vi "Drivetrain.vi"() -> ()   [LabVIEW 2012]
uses:
  <vilib>/Rock Robotics/WPI/Solenoid/WPI_SolenoidValue.ctl
  Robot Global Data.vi
  <vilib>/Rock Robotics/WPI/RobotDrive/WPI_RobotDriveGetSetRefNum.vi
  <vilib>/addons/control/pid/NI_PID_pid.lvlib
  <vilib>/addons/control/pid/pid.llb/PID (DBL).vi
panel:
  in  "PID gains":T1={"proportional gain (Kc)"=20.0, "integral time (Ti, min)"=0.008, "derivative time (Td, min)"=0.001} {"derivative time (Td, min)" format="%.3f"; "integral time (Ti, min)" format="%.3f"; "proportional gain (Kc)" format="%.3f"}
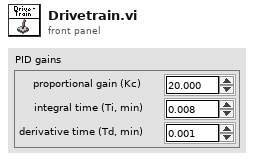
[diagram p1: front panel]
types:
  T1 = cluster{"proportional gain (Kc)":dbl, "integral time (Ti, min)":dbl, "derivative time (Td, min)":dbl}
  T2 = typedef "WPI_SolenoidValue.ctl" = enum16{"Off", "On", "Forward", "Reverse"}
  T3 = typedef "WPI_RelayDevRef.ctl" = cluster{"DevStatus":errorcluster, "Relay Channel":T4, "Digital Module":T5, "Relay Direction":T6}
  T4 = typedef "FPGA_DIORelayChannel.ctl" = enum8{"Relay 1", "Relay 2", "Relay 3", "Relay 4", "Relay 5", "Relay 6", "Relay 7", "Relay 8", "Invalid"}
  T5 = typedef "FPGA_TypedefDigitalModule.ctl" = enum16{"Digital Module 1", "Digital Module 2"}
  T6 = typedef "WPI_RelayDirection.ctl" = enum16{"Both directions", "Forward only", "Reverse only"}
  T7 = typedef "WPI_RobotDriveDevRef.ctl" = cluster{"DevStatus":errorcluster, "Motors[]":T8[], "Square Inputs":bool, "Max Output":dbl, "Isochronous":bool}
  T8 = typedef "WPI_MotorControlDeviceRef.ctl" = cluster{"DeviceStatus":errorcluster, "Type":enum16{"PWM", "CAN"}, "PWM":cluster{"Digital Module":T5, "PWM Channel":T9, "DeadBand":T10}, "CAN":cluster{"Device Number":u8, "Control Mode":T11, "Semaphore":T12, "Max Vout":dbl}, "Invert":bool, "TransformRef":T13, "InvTransformRef":T13}
  T9 = typedef "FPGA_DIOPWMChannel.ctl" = enum8{"PWM 1", "PWM 2", "PWM 3", "PWM 4", "PWM 5", "PWM 6", "PWM 7", "PWM 8", "PWM 9", "PWM 10", "Invalid"}
  T10 = typedef "WPI_PWMDeadband.ctl" = cluster{"Name":string, "maxPositivePwm":i32, "minPositivePwm":i32, "centerPwm":i32, "maxNegativePwm":i32, "minNegativePwm":i32, "angularRange":u16}
  T11 = typedef "WPI_CANJaguar_ControlMode.ctl" = enum8{"Percent VBus", "Current", "Speed", "Position", "Voltage"}
  T12 = typedef "Semaphore RefNum" = refnum<k1>
  T13 = typedef "WPI_PWMTransform_ConPane.ctl" = refnum<vi>
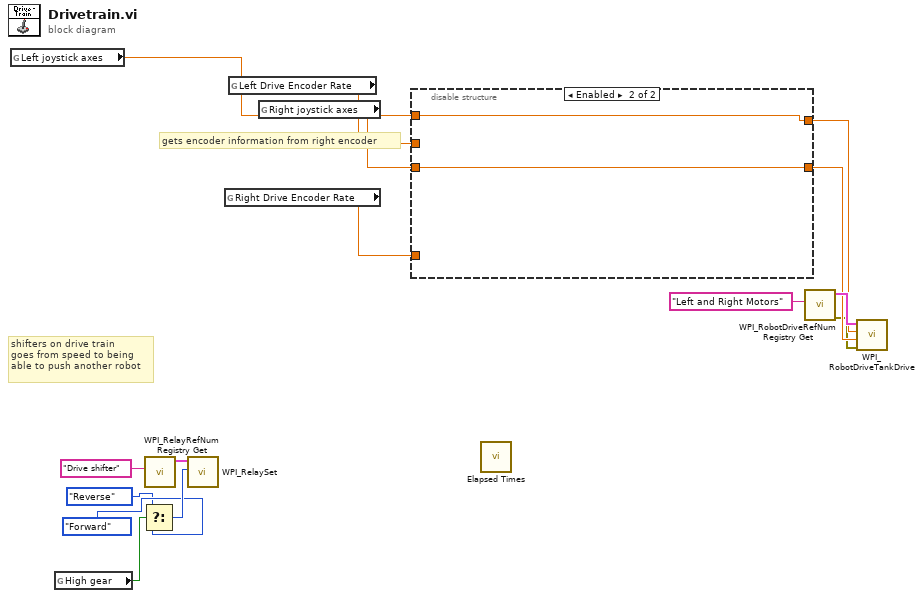
[diagram p0: block diagram]
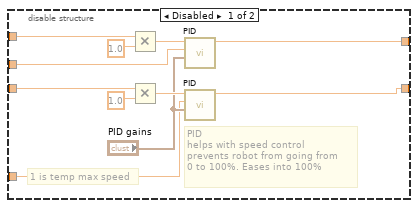
[diagram p2: hidden frame]
diagram:
  # "shifters on drive train\ngoes from speed to being\nable to push another robot"
  # "gets encoder information from right encoder"
  n1 = global read "Robot Global Data.vi" "Left joystick axes"() -> (w8:dbl)
  n2 = global read "Robot Global Data.vi" "High gear"() -> (w5:bool)
  n3 = Select(t=WPI_SolenoidValue."Reverse" ("Value"), s=w5, f=WPI_SolenoidValue."Forward" ("Value")) -> (s? t:f=w6:T2)
  n4 = call <vilib>:"WPI_RelayRefNum Registry Get.vi"("refnum name"="Drive shifter") -> ("RelayDevRef"=w2:T3)  [unwired: 9 in, 1 out]
  n5 = call <vilib>:"WPI_RelaySet.vi"("RelayValue"=w6, "RelayDevRef"=w2) -> ()  [unwired: 8 in, 2 out]
  n6 = global read "Robot Global Data.vi" "Right Drive Encoder Rate"() -> (w13:dbl)
  n7 = global read "Robot Global Data.vi" "Left Drive Encoder Rate"() -> (w12:dbl)
  n8 = global read "Robot Global Data.vi" "Right joystick axes"() -> (w7:dbl)
  n9 = disable-structure shown="Enabled" {
    disable-tunnel: w8 -> [w25 w28]
    disable-tunnel: [w23 w28] -> w11
    disable-tunnel: w12 -> [w22 _]
    disable-tunnel: [w18 w27] -> w10
    disable-tunnel: w13 -> [w17 _]
    disable-tunnel: w7 -> [w16 w27]
    frame Disabled {
      # "1 is temp max speed"
      # "PID\nhelps with speed control \nprevents robot from going from\n0 to 100%. Eases into 100%"
      n10 = Multiply(x=w25, y=1.0) -> (x*y=w24:dbl)
      n11 = Multiply(x=w16, y=1.0) -> (x*y=w20:dbl)
      n12 = call-poly <vilib>:"PID.vi"("PID gains"="PID gains", "process variable"=w22, "setpoint"=w24) -> ("output"=w23:dbl)  [unwired: 7 in, 1 out]
      n13 = call-poly <vilib>:"PID.vi"("PID gains"="PID gains", "process variable"=w17, "setpoint"=w20) -> ("output"=w18:dbl)  [unwired: 7 in, 1 out]
    }
    frame Enabled {
    }
  }
  n14 = call "Elapsed Times.vi"() -> ()  [unwired: 3 in, 1 out]
  n15 = call <vilib>:"WPI_RobotDriveRefNum Registry Get.vi"("refnum name"="Left and Right Motors") -> ("error out"=w9:errorcluster, "RobotDriveDevRef"=w15:T7)  [unwired: 1 in, 8 out]
  n16 = call <vilib>:"WPI_RobotDriveTankDrive.vi"("error in (no error)"=w9, "Right axis value"=w10, "Left axis value"=w11, "RobotDriveDevRef"=w15) -> ()  [unwired: 5 in, 3 out]
